vi "Read Slidebook Parameters File.vi"(8 "error in (no error)":errorcluster, 11 "SPCParameters IN":T1) -> (0 "error out":errorcluster, 1 "New File?":bool, 2 "Dwell Time (us)":dbl, 3 "SPCParameters OUT":T1)   [LabVIEW 2016]
uses:
  SPCParameters Control.ctl
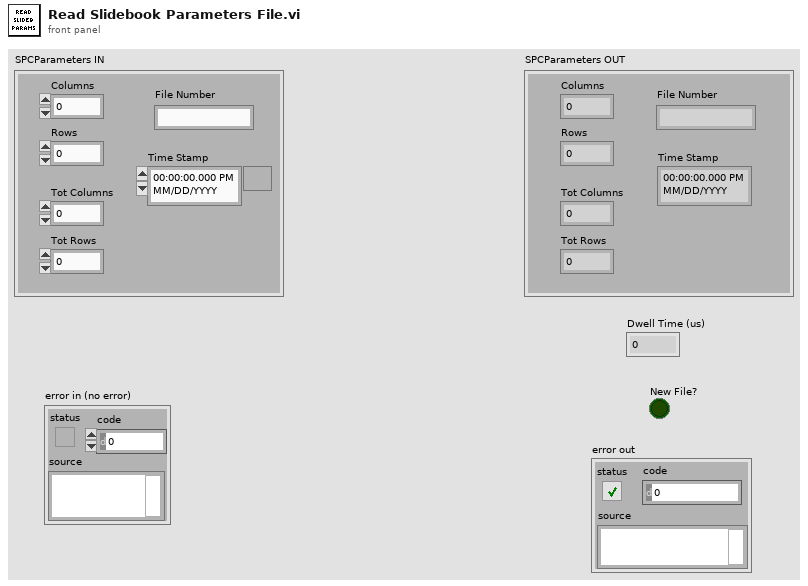
[diagram p1: front panel]
types:
  T1 = typedef "SPCParameters Control.ctl" = cluster{"Columns":u16, "Rows":u16, "Tot Columns":u16, "Tot Rows":u16, "File Number":string, "Time Stamp":timestamp}
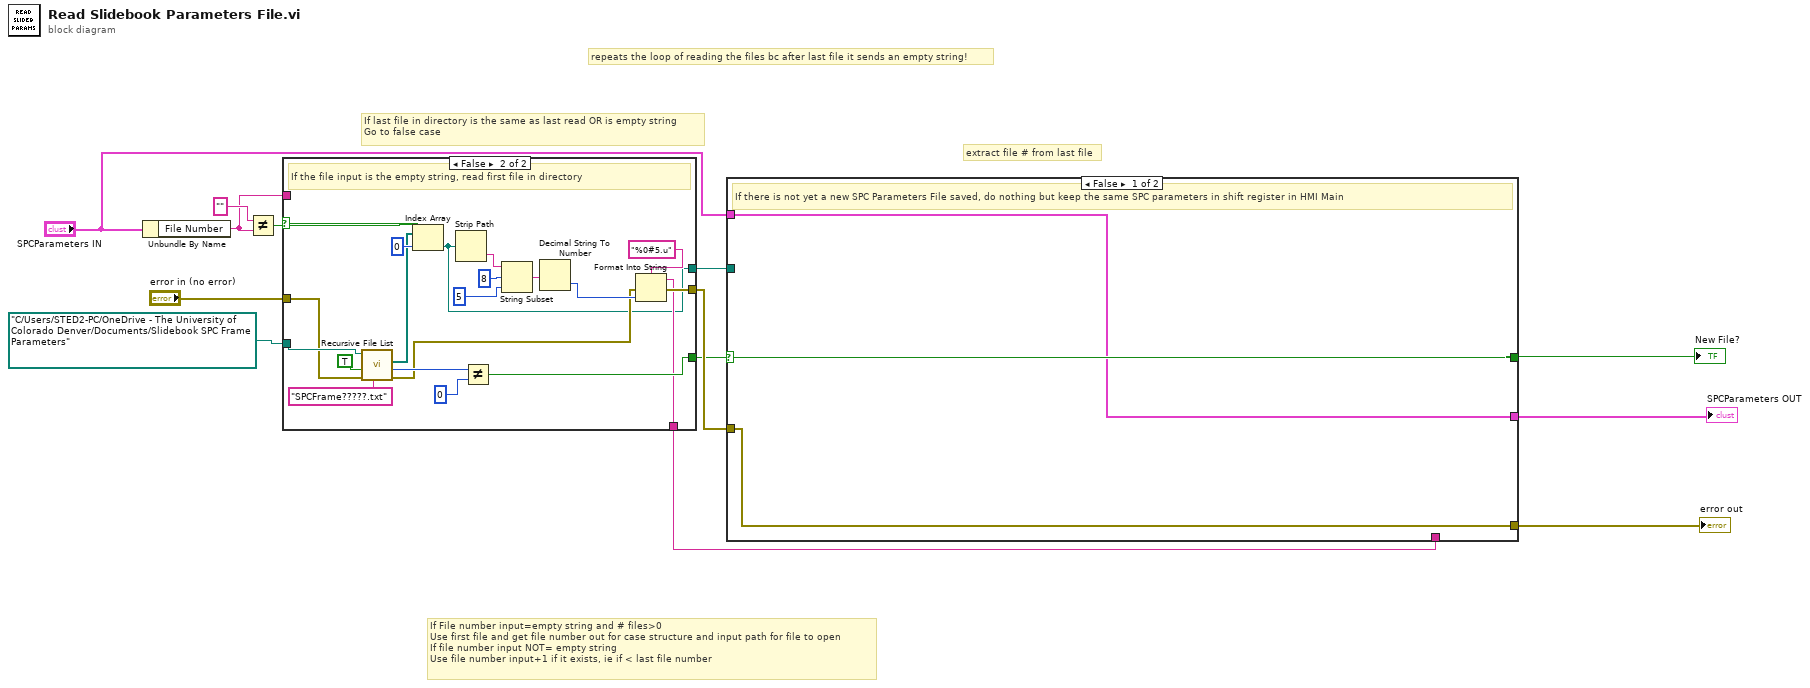
[diagram p0: block diagram]
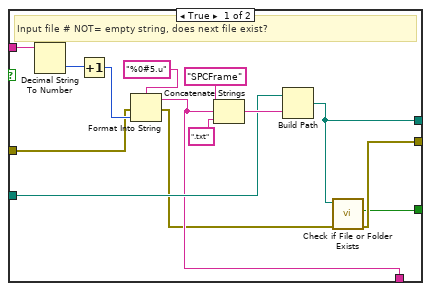
[diagram p2: hidden frame]
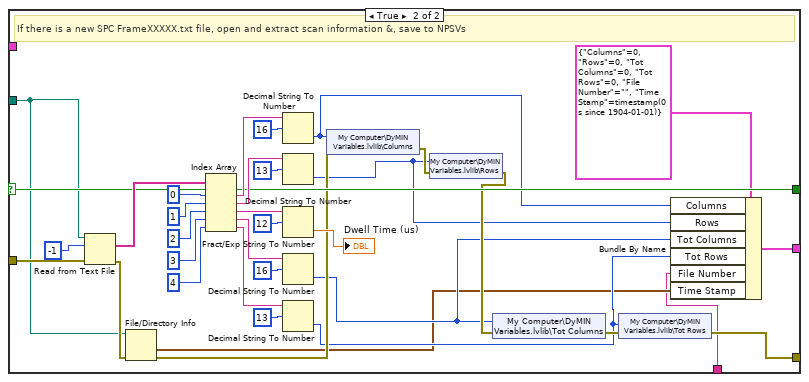
[diagram p3: hidden frame]
diagram:
  # "repeats the loop of reading the files bc after last file it sends an empty string!"
  # "If File number input=empty string and # files>0\nUse first file and get file number out for case structure and input path for file to open\nIf file number input NOT= empty string\nUse file number input+1 if it exists, ie if < last file number"
  # "extract file # from last file"
  # "If last file in directory is the same as last read OR is empty string\nGo to false case"
  n1 = Unbundle By Name("SPCParameters IN") -> ("File Number"=w9:string)
  n2 = Not Equal?(x="", y=w9) -> (x != y?=w8:bool)
  n3 = case shown="False" w8 {
    tunnel: w9 -> [w26 _]
    tunnel: "error in (no error)" -> [w23 w35]
    tunnel: path "C:/Users/STED2-PC/OneDrive - The University of Colorado Denver/Documents/Slidebook SPC Frame Parameters" ("Folder Path") -> [w19 w39]
    tunnel: [w14 w34] -> w4
    tunnel: [w15 w30] -> w5
    tunnel: [w18 w29] -> w2
    tunnel: [w17 w28] -> w3
    frame True {
      # "Input file # NOT= empty string, does next file exist?"
      n4 = Decimal String To Number(string=w26) -> (number=w27:i32)  [unwired: 2 in, 1 out]
      n5 = Increment(x=w27) -> (x+1=w24:i32)
      n6 = Format Into String(format string="%0#5.u", error in=w23, w24) -> (resulting string=w18:string, error out=w16:errorcluster)  [unwired: 1 in]
      n7 = Concatenate Strings("SPCFrame" ("string"), w18, ".txt" ("string")) -> (w21:string)
      n8 = Build Path(base path=w19, name or relative path=w21) -> (appended path=w17:path)
      n9 = call <vilib>:"Check if File or Folder Exists.vi"("error in (no error)"=w16, "path"=w17) -> ("error out"=w15:errorcluster, "file or folder exists?"=w14:bool)  [unwired: 7 in, 1 out]
    }
    frame False {
      # "If the file input is the empty string, read first file in directory"
      n10 = call <vilib>:"Recursive File List.vi"("pattern"="SPCFrame?????.txt", "error in (no error)"=w35, "Continue Recursing on Error? (F)"=TRUE, "Folder Path"=w39) -> ("error out"=w31:errorcluster, "Number of Files"=w36:i32, "All Files in Dir"=w38:path[])  [unwired: 3 in, 2 out]
      n11 = Index Array(array=w38, index=0) -> (element=w28:path)
      n12 = Strip Path(path=w28) -> (name=w46:string)  [unwired: 1 out]
      n13 = Not Equal?(x=w36, y=0) -> (x != y?=w34:bool)
      n14 = String Subset(string=w46, offset (0)=8, length (rest)=5 ("length (rest)")) -> (substring=w43:string)
      n15 = Decimal String To Number(string=w43) -> (number=w33:i32)  [unwired: 2 in, 1 out]
      n16 = Format Into String(format string="%0#5.u", error in=w31, w33) -> (resulting string=w29:string, error out=w30:errorcluster)  [unwired: 1 in]
    }
  }
  n17 = case shown="False" w4 {
    selector: w4 -> [w49 w66]
    tunnel: [w48 w60] -> w13
    tunnel: [w49 w66] -> w12
    tunnel: [w47 w53] -> w11
    tunnel: w5 -> [w48 w52]
    tunnel: w3 -> [_ w50]
    tunnel: w2 -> [_ w51]
    tunnel: "SPCParameters IN" -> [w47 _]
    frame False {
      # "If there is not yet a new SPC Parameters File saved, do nothing but keep the same SPC parameters in shift register in HMI Main"
    }
    frame True {
      # "If there is a new SPC FrameXXXXX.txt file, open and extract scan information &, save to NPSVs"
      n18 = Read from Text File(file (use dialog)=w50, count=-1, error in=w52) -> (text=w83:string[], error out=w65:errorcluster)  [unwired: 1 in, 2 out]
      n19 = File/Directory Info(path=w50, error in=w65) -> (last mod=w54:timestamp, error out=w64:errorcluster)  [unwired: 5 out]
      n20 = Index Array(array=w83, index #1=0 ("index"), index #2=1 ("index"), index #3=2 ("index"), index #4=3 ("index"), index #5=4 ("index")) -> (element #1=w77:string, element #2=w73:string, element #3=w75:string, element #4=w71:string, element #5=w69:string)
      n21 = Decimal String To Number(string=w77, offset=16 ("offset (0)")) -> (number=w58:i32)  [unwired: 1 in, 1 out]
      n22 = Decimal String To Number(string=w73, offset=13 ("offset (0)")) -> (number=w57:i32)  [unwired: 1 in, 1 out]
      n23 = Fract/Exp String To Number(string=w75, offset=12 ("offset (0)")) -> (number=→"Dwell Time (us)":dbl)  [unwired: 2 in, 1 out]
      n24 = Decimal String To Number(string=w71, offset=16 ("offset (0)")) -> (number=w56:i32)  [unwired: 1 in, 1 out]
      n25 = Decimal String To Number(string=w69, offset=13 ("offset (0)")) -> (number=w55:i32)  [unwired: 1 in, 1 out]
      n26 = shared-variable "My Computer\\DyMIN Variables.lvlib\\Columns"(w58, error in=w64) -> (error out=w63:errorcluster)
      n27 = shared-variable "My Computer\\DyMIN Variables.lvlib\\Rows"(w57, error in=w63) -> (error out=w62:errorcluster)
      n28 = shared-variable "My Computer\\DyMIN Variables.lvlib\\Tot Columns"(w56, error in=w62) -> (error out=w61:errorcluster)
      n29 = shared-variable "My Computer\\DyMIN Variables.lvlib\\Tot Rows"(w55, error in=w61) -> (error out=w60:errorcluster)
      n30 = Bundle By Name(cluster=T1 {"Columns"=0, "Rows"=0, "Tot Columns"=0, "Tot Rows"=0, "File Number"="", "Time Stamp"=timestamp(0 s since 1904-01-01)} ("SPCParameters 2"), "Columns"=w58, "Rows"=w57, "Tot Columns"=w56, "Tot Rows"=w55, "File Number"=w51, "Time Stamp"=w54) -> (w53:T1)
    }
  }
  "error out" <- w13
  "New File?" <- w12
  "SPCParameters OUT" <- w11
